vi "CS-4 Setup Dialog.vi"(8 "error in":errorcluster, 11 "VISA session":refnum<visa-resource-name>) -> (0 "error out":errorcluster, 1 "sweep rates out":T1 {"rate 3" format="%.2f"; "rate 2" format="%.2f"; "rate 1" format="%.2f"; "rate 0" format="%.2f"}, 2 "sweep range":cluster{"range 0":dbl, "range 1":dbl}={"range 0"=60.0, "range 1"=85.0} {"range 1" format="%.3f"; "range 0" format="%.3f"}, 3 "dup VISA session":refnum<visa-resource-name>, 4 "send":bool, 5 "limits out":T2 {"Voltage Limit" format="%.2f"; "Upper Current Limit" format="%.2f"; "Lower Current Limit" format="%.2f"}, 7 "Units":enum16{"Amps", "Kilogauss", "Tesla"}(ring))   [LabVIEW 2016]
doc: "CS-4 Setup.vi is implemented as a dialog that uses CS-4 Recall.vi to recall present CS-4 parameters, and CS-4 Config.vi to update the supply with new charge rates and limits. Logic is simplified by requiring that Units be changed elsewhere.\n\nA VISA channel must be opened using CS-4 Initialize.vi before this VI is invoked."
panel:
  out "min supply current":dbl=100.0 format="%.3f"
  in  "range 1":dbl=85.0 min=0.0 max=1000.0 format="%.3f"
  in  "range 0":dbl=60.0 min=0.0 max=1000.0 format="%.3f"
  in  "limits":T2={"Lower Current Limit"=-10.0, "Upper Current Limit"=10.0, "Voltage Limit"=5.0} {"Voltage Limit" min=0.0 max=5.0 format="%.2f"; "Upper Current Limit" min=-1000.0 max=1000.0 format="%.2f"; "Lower Current Limit" min=-1000.0 max=1000.0 format="%.1f"}
  in  "sweep rates":T1={"rate 0"=0.5, "rate 1"=0.25, "rate 2"=0.1, "rate 3"=10.0} {"rate 3" min=0.0 max=100.0 step=0.0001 format="%.4f"; "rate 2" min=0.0 max=100.0 step=0.0001 format="%.4f"; "rate 1" min=0.0 max=100.0 step=0.0001 format="%.4f"; "rate 0" min=0.0 max=100.0 step=0.0001 format="%.4f"}
  in  "Cancel":bool
  in  "Send":bool
  out "max supply current":dbl=100.0 format="%.3f"
  out "range 2 start":dbl format="%.3f"
  out "range 1 start":dbl format="%.3f"
  # "Model CS-4 Magnet Power Supply Setup"
  # "Sweep Rates"
  # "Range 1"
  # "0.000"
  # "TO"
  # "Range 2"
  # "TO"
  # "Range 3"
  # "TO"
  # "Fast Mode"
  # "Limits"
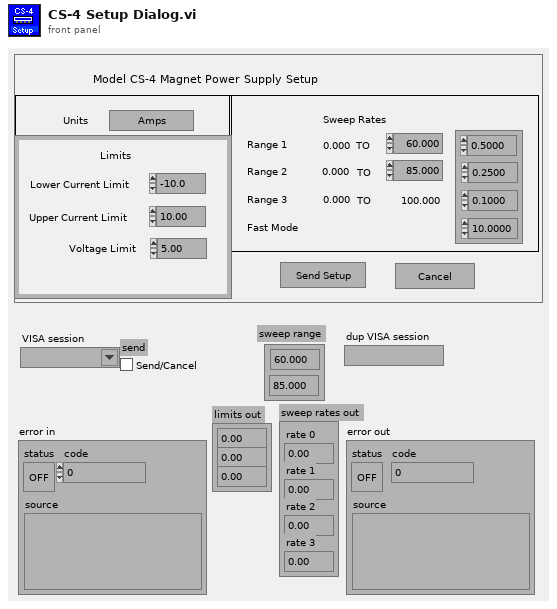
[diagram p1: front panel]
types:
  T1 = cluster{"rate 0":dbl, "rate 1":dbl, "rate 2":dbl, "rate 3":dbl}
  T2 = cluster{"Lower Current Limit":dbl, "Upper Current Limit":dbl, "Voltage Limit":dbl}
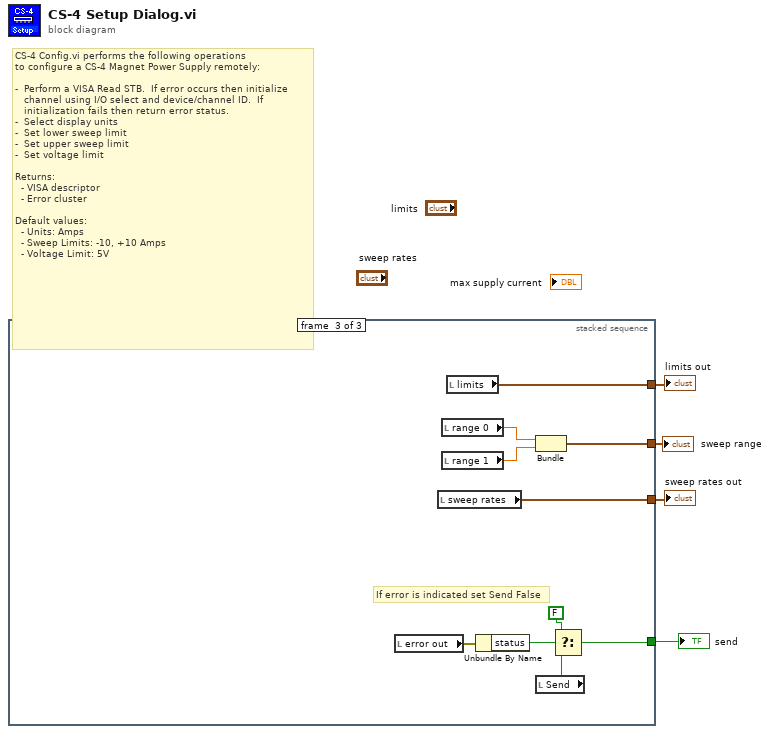
[diagram p0: block diagram]
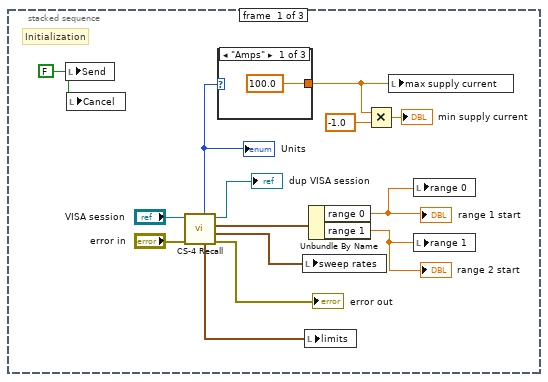
[diagram p2: hidden frame]
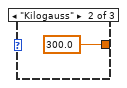
[diagram p3: hidden frame]
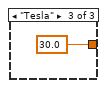
[diagram p4: hidden frame]
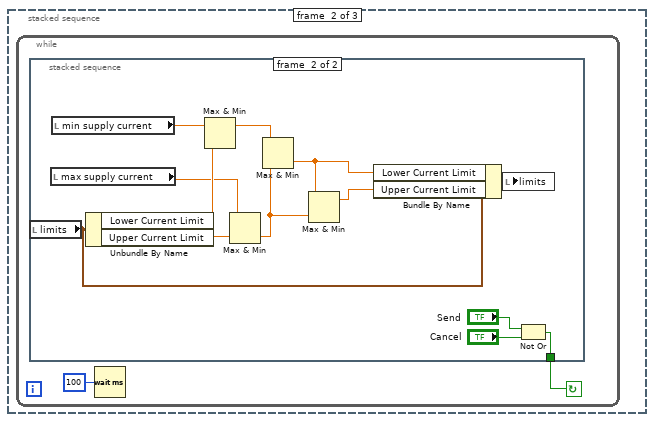
[diagram p5: hidden frame]
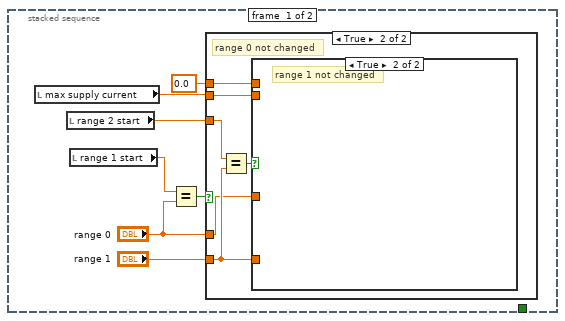
[diagram p6: hidden frame]
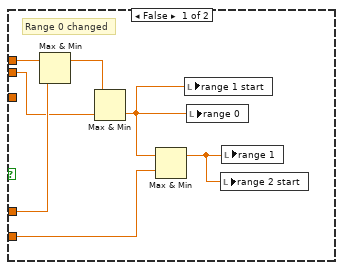
[diagram p7: hidden frame]
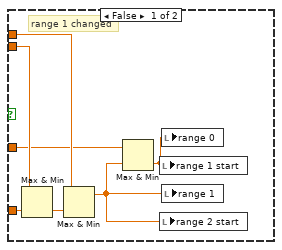
[diagram p8: hidden frame]
diagram:
  # "CS-4 Config.vi performs the following operations\nto configure a CS-4 Magnet Power Supply remotely:\n\n-  Perform a VISA Read STB.  If error occurs then initialize \n   channel using I/O select and device/channel ID.  If \n   initialization fails then return error status.\n-  Select display units\n-  Set lower sweep limit\n-  Set upper sweep limit\n-  Set voltage limit\n\nReturns:\n  - VISA descriptor\n  - Error cluster\n\nDefault values:\n  - Units: Amps\n  - Sweep Limits: -10, +10 Amps\n  - Voltage Limit: 5V"
  n1 = stacked-sequence {
    tunnel: [_ _ w67] -> w4
    tunnel: [_ _ w66] -> w3
    tunnel: [_ _ w65] -> w2
    tunnel: [_ _ w64] -> w1
    frame #0 {
      w18 = FALSE ("Send")
      # "Initialization"
      n2 = local write "Send"(w18) -> ()
      n3 = local write "Cancel"(w18) -> ()
      n4 = call "CS-4 Recall.vi"("error in (no error)"="error in", "VISA session"="VISA session") -> ("error out"=→"error out":errorcluster, "sweep rates"=w9:T1, "range"=w13:cluster{"range 0":dbl, "range 1":dbl}, "dup VISA session"=→"dup VISA session":refnum<visa-resource-name>, "limits"=w10:T2, "Units"=w5:enum16{"Amps", "Kilogauss", "Tesla"})  [unwired: 4 in]
      "Units" <- w5
      n5 = case shown="\"Amps\"" w5 {
        tunnel: [100.0 ("max supply current") 300.0 ("max supply current") 30.0 ("max supply current")] -> w6
        frame "Amps" {
        }
        frame "Kilogauss" {
        }
        frame "Tesla" {
        }
      }
      n6 = local write "sweep rates"(w9) -> ()
      n7 = local write "limits"(w10) -> ()
      n8 = Unbundle By Name(w13) -> ("range 0"=w12:dbl, "range 1"=w11:dbl)
      "range 1 start" <- w12
      "range 2 start" <- w11
      n9 = Multiply(x=w6, y=-1.0) -> (x*y=→"min supply current":dbl)
      n10 = local write "max supply current"(w6) -> ()
      n11 = local write "range 0"(w12) -> ()
      n12 = local write "range 1"(w11) -> ()
    }
    frame #1 {
      n13 = while {
        stop <- w22 continue-if-true
        n14 = stacked-sequence {
          tunnel: [_ w51] -> w22
          frame #0 {
            n15 = local read "max supply current"() -> (w25:dbl)
            n16 = local read "range 2 start"() -> (w29:dbl)
            n17 = local read "range 1 start"() -> (w26:dbl)
            n18 = Equal?(x=w26, y="range 0") -> (x = y?=w27:bool)
            n19 = case shown="True" w27 {
              tunnel: "range 1" -> [w33 w41]
              tunnel: w29 -> [_ w43]
              tunnel: w25 -> [w35 w40]
              tunnel: "range 0" -> [w36 w39]
              tunnel: 0.0 -> [w37 w38]
              frame False {
                # "Range 0 changed"
                n20 = Max & Min(x=w37, y=w36) -> (max(x,y)=w34:dbl)  [unwired: 1 out]
                n21 = Max & Min(x=w34, y=w35) -> (min(x,y)=w32:dbl)  [unwired: 1 out]
                n22 = Max & Min(x=w32, y=w33) -> (max(x,y)=w31:dbl)  [unwired: 1 out]
                n23 = local write "range 1 start"(w32) -> ()
                n24 = local write "range 0"(w32) -> ()
                n25 = local write "range 2 start"(w31) -> ()
                n26 = local write "range 1"(w31) -> ()
              }
              frame True {
                # "range 0 not changed"
                n27 = Equal?(x=w43, y=w41) -> (x = y?=w42:bool)
                n28 = case shown="True" w42 {
                  tunnel: w41 -> [w50 _]
                  tunnel: w40 -> [w49 _]
                  tunnel: w39 -> [w46 _]
                  tunnel: w38 -> [w47 _]
                  frame False {
                    # "range 1 changed"
                    n29 = Max & Min(x=w49, y=w50) -> (min(x,y)=w48:dbl)  [unwired: 1 out]
                    n30 = Max & Min(x=w47, y=w48) -> (max(x,y)=w45:dbl)  [unwired: 1 out]
                    n31 = Max & Min(x=w46, y=w45) -> (min(x,y)=w44:dbl)  [unwired: 1 out]
                    n32 = local write "range 1 start"(w44) -> ()
                    n33 = local write "range 2 start"(w45) -> ()
                    n34 = local write "range 0"(w44) -> ()
                    n35 = local write "range 1"(w45) -> ()
                  }
                  frame True {
                    # "range 1 not changed"
                  }
                }
              }
            }
          }
          frame #1 {
            n36 = local read "limits"() -> (w60:T2)
            n37 = local read "max supply current"() -> (w59:dbl)
            n38 = local read "min supply current"() -> (w61:dbl)
            n39 = Unbundle By Name(w60) -> ("Lower Current Limit"=w63:dbl, "Upper Current Limit"=w62:dbl)
            n40 = Max & Min(x=w61, y=w63) -> (max(x,y)=w55:dbl)  [unwired: 1 out]
            n41 = Max & Min(x=w59, y=w62) -> (min(x,y)=w57:dbl)  [unwired: 1 out]
            n42 = Max & Min(x=w55, y=w57) -> (min(x,y)=w54:dbl)  [unwired: 1 out]
            n43 = Max & Min(x=w54, y=w57) -> (max(x,y)=w56:dbl)  [unwired: 1 out]
            n44 = Bundle By Name(cluster=w60, "Lower Current Limit"=w54, "Upper Current Limit"=w56) -> (w58:T2)
            n45 = local write "limits"(w58) -> ()
            n46 = Not Or(1:"Cancel", 2:"Send") -> (0:w51:bool)
          }
        }
        n47 = Wait (ms)(milliseconds to wait=u32 100) -> ()  [unwired: 1 out]
      }
    }
    frame #2 {
      # "If error is indicated set Send False"
      n48 = local read "error out"() -> (w71:errorcluster)
      n49 = local read "sweep rates"() -> (w64:T1)
      n50 = local read "range 0"() -> (w73:dbl)
      n51 = local read "range 1"() -> (w72:dbl)
      n52 = local read "limits"() -> (w65:T2)
      n53 = Unbundle By Name(w71) -> ("status"=w69:bool)
      n54 = Bundle("range 0"=w73, "range 1"=w72) -> (w67:cluster{"range 0":dbl, "range 1":dbl})  [unwired: 1 in]
      n55 = local read "Send"() -> (w70:bool)
      n56 = Select(t=FALSE, s=w69, f=w70) -> (s? t:f=w66:bool)
    }
  }
  "sweep range" <- w4
  "send" <- w3
  "limits out" <- w2
  "sweep rates out" <- w1
